vi "std sort simple.vi"(8 "error in":errorcluster, 11 "cycle results cluster IN":T2) -> (0 "error out":errorcluster, 3 "output cluster":T1)   [LabVIEW 2016]
uses:
  controls/cycle results control.ctl
  controls/data control cluster.ctl
panel:
  out "Array 2":dbl[][](array[numeric])
  out "Array":dbl[][][](array[numeric])
  out "element 2":dbl
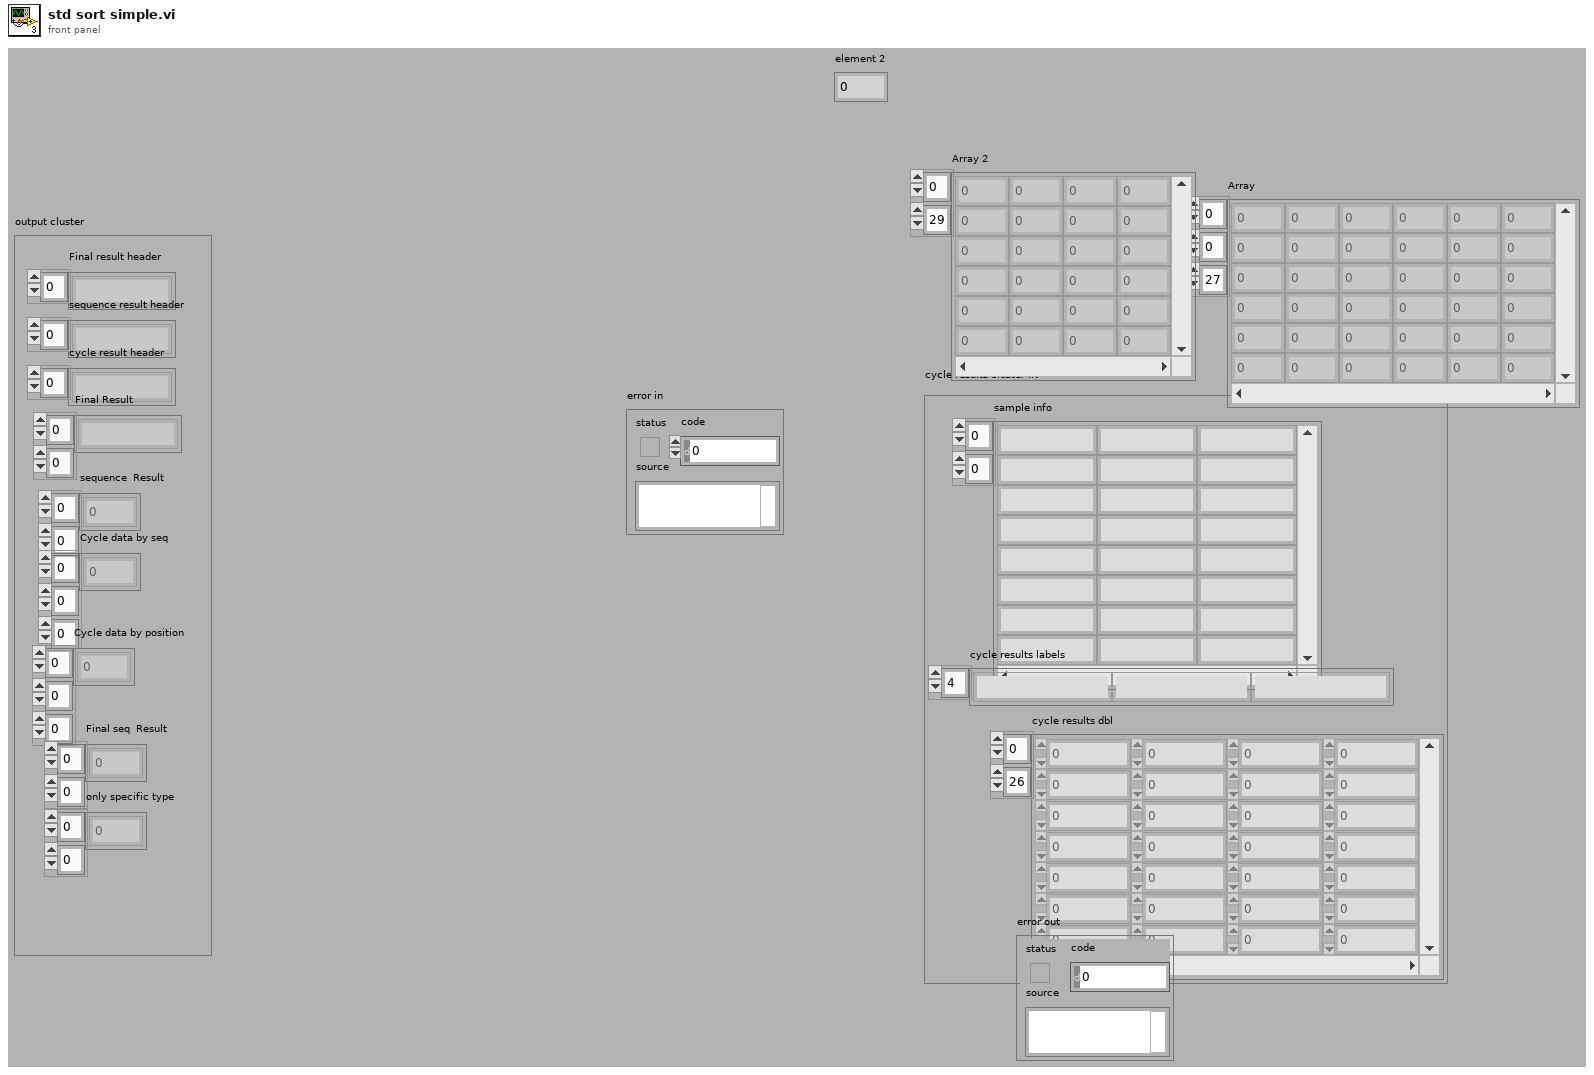
[diagram p1: front panel]
types:
  T1 = typedef "data control cluster.ctl" = cluster{"Final result header":string[], "sequence result header":string[], "cycle result header ":string[], "Final Result":string[][], "sequence  Result":dbl[][], "Cycle data by seq":dbl[][][], "Cycle data by position":dbl[][][], "Final seq  Result":dbl[][], "only specific type":dbl[][]}
  T2 = typedef "cycle results control.ctl" = cluster{"sample info":string[][], "cycle results labels":string[], "cycle results dbl":dbl[][]}
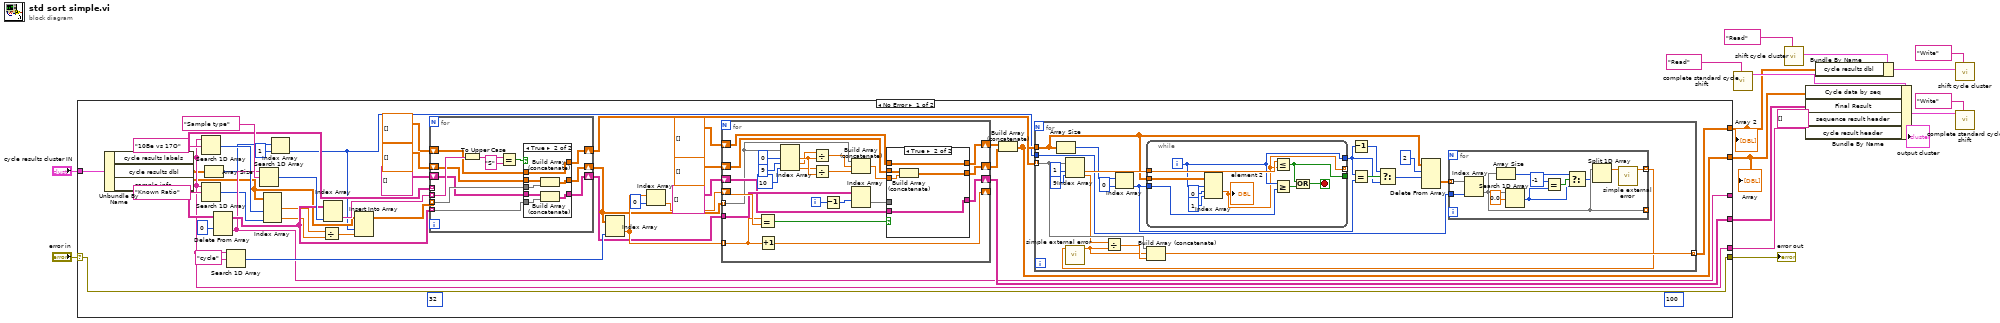
[diagram p0: block diagram]
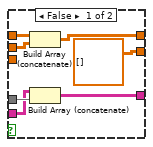
[diagram p2: hidden frame]
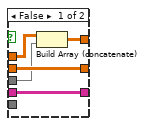
[diagram p3: hidden frame]
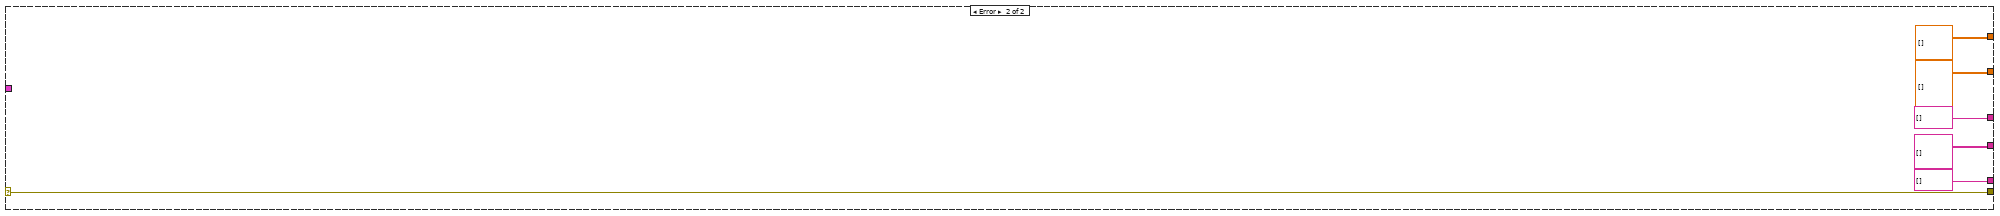
[diagram p4: hidden frame]
diagram:
  n1 = case shown="No Error" "error in" {
    selector: "error in" -> [w57 w164]
    tunnel: "cycle results cluster IN" -> [w35 _]
    tunnel: [w57 w164] -> w14
    tunnel: [w37 string[][] []] -> w7
    tunnel: [w36 string[] [] ("sample info")] -> _
    tunnel: [w19 dbl[][][] []] -> w6
    tunnel: [w32 string[] [] ("cycle results labels")] -> w9
    tunnel: [w17 dbl[][] []] -> w2
    frame No Error {
      (unwired) 32
      (unwired) 100 ("disabled index (col)")
      n2 = Unbundle By Name(w35) -> ("cycle results labels"=w32:string[], "cycle results dbl"=w25:dbl[][], "sample info"=w51:string[][])
      n3 = Search 1D Array(1D array=w32, element="10Be vs 17O") -> (index of element=w31:i32)  [unwired: 1 in]
      n4 = Search 1D Array(1D array=w32, element="Known Ratio") -> (index of element=w30:i32)  [unwired: 1 in]
      n5 = Array Size(array=w25) -> (size(s)=w24:i32[])
      n6 = Delete From Array(array=w51, index (row)=0) -> (deleted portion=w36:string[], array with subset deleted=w50:string[][])  [unwired: 2 in]
      n7 = Search 1D Array(1D array=w32, element="cycle") -> (index of element=w47:i32)  [unwired: 1 in]
      n8 = Search 1D Array(1D array=w36, element="Sample type") -> (index of element=w54:i32)  [unwired: 1 in]
      n9 = Index Array(array=w25, index (col) #1=w31, index (col) #2=w30) -> (element #1=w29:dbl[], element #2=w28:dbl[])  [unwired: 2 in]
      n10 = Index Array(array=w24, index=1) -> (element=w18:i32)
      n11 = Divide(x=w29, y=w28) -> (x/y=w26:dbl[])
      n12 = Index Array(array=w50, index (col)=w54) -> (element=w53:string[])  [unwired: 1 in]
      n13 = Insert Into Array(array=w25, index (col)=w18, new element=w26) -> (w27:dbl[][])  [unwired: 1 in]
      n14 = for {
        tunnel: w51 -> [_] mode=indexing
        tunnel: w27 -> [w142] mode=indexing
        tunnel: w53 -> [w146] mode=indexing
        shift-right: [w141] -> w21
        shift-left: dbl[][] [] -> [w140]
        tunnel: w50 -> [w139] mode=indexing
        shift-right: [w138] -> w39
        shift-left: string[][] [] -> [w137]
        shift-right: [w136] -> w20
        shift-left: dbl[][] [] -> [w135]
        n15 = To Upper Case(1:w146) -> (0:w145:string)
        n16 = Equal?(x=w145, y="S") -> (x = y?=w143:bool)
        n17 = case shown="True" w143 {
          tunnel: w142 -> [w149 w158]
          tunnel: [w151 w157] -> w141
          tunnel: w140 -> [w151 w156]
          tunnel: w139 -> [_ w155]
          tunnel: [w150 w153] -> w138
          tunnel: w137 -> [w150 w154]
          tunnel: [w148 w152] -> w136
          tunnel: w135 -> [w147 w152]
          frame False {
            n18 = Build Array (concatenate)(w147, w149) -> (w148:dbl[][])
          }
          frame True {
            n19 = Build Array (concatenate)(w156, w158) -> (w157:dbl[][])
            n20 = Build Array (concatenate)(w154, w155) -> (w153:string[][])
          }
        }
      }
      n21 = Index Array(array=w21, index (col)=w47) -> (element=w46:dbl[])  [unwired: 1 in]
      n22 = Index Array(array=w46, index=0) -> (element=w40:dbl)
      n23 = for {
        tunnel: w46 -> [w116] mode=indexing
        shift-right: [w115] -> _
        shift-left: w40 -> [w122]
        tunnel: w21 -> [w102] mode=indexing
        shift-right: [w121] -> w43
        shift-left: dbl[][] [] -> [w120]
        shift-right: [w119] -> w42
        shift-left: dbl[][][] [] -> [w118]
        tunnel: w39 -> [w114]
        shift-right: [w112] -> w37
        shift-left: string[][] [] -> [w110]
        i -> [w113]
        n24 = Equal?(x=w116, y=w122) -> (x = y?=w117:bool)
        n25 = Increment(x=w116) -> (x+1=w115:dbl)
        n26 = Index Array(array=w102, index #1=0 ("index"), index #2=9 ("index"), index #3=10 ("index")) -> (element #1=w105:dbl, element #2=w103:dbl, element #3=w104:dbl)
        n27 = Divide(x=w103, y=w105) -> (x/y=w101:dbl)
        n28 = Divide(x=w104, y=w105) -> (x/y=w100:dbl)
        n29 = Decrement(x=w113) -> (x-1=w109:i32)
        n30 = Build Array (concatenate)(w102, w101, w100) -> (w99:dbl[])
        n31 = Index Array(array=w114, index (row)=w109) -> (element=w111:string[])  [unwired: 1 in]
        n32 = case shown="True" w117 {
          tunnel: w99 -> [_ w134]
          tunnel: [dbl[][] [] w133] -> w121
          tunnel: w120 -> [w129 w132]
          tunnel: [w128 w131] -> w119
          tunnel: w118 -> [w127 w131]
          tunnel: [w123 w130] -> w112
          tunnel: w111 -> [w125 _]
          tunnel: w110 -> [w124 w130]
          frame False {
            n33 = Build Array (concatenate)(w127, w129) -> (w128:dbl[][][])
            n34 = Build Array (concatenate)(w124, w125) -> (w123:string[][])
          }
          frame True {
            n35 = Build Array (concatenate)(w132, w134) -> (w133:dbl[][])
          }
        }
      }
      n36 = Build Array (concatenate)(w42, w43) -> (w19:dbl[][][])
      n37 = for {
        tunnel: w20 -> [w68] mode=indexing
        tunnel: w19 -> [w72]
        tunnel: w18 -> [w69]
        tunnel: [w67] -> w17 mode=indexing
        n38 = Array Size(array=w72) -> (size(s)=w74:i32[])
        n39 = Index Array(array=w68, index #1=1 ("index"), index #2=9 ("index")) -> (element #1=w75:dbl, element #2=w64:dbl)
        n40 = Index Array(array=w74, index=0) -> (element=w63:i32)
        n41 = while {
          tunnel: w72 -> [w98]
          tunnel: w75 -> [w95]
          tunnel: w63 -> [w94]
          tunnel: [w91] -> w60
          tunnel: [w90] -> _
          tunnel: [w89] -> _ mode=indexing
          i -> [w91]
          stop <- w92 stop-if-true
          n42 = Index Array(array=w98, index (dim 0)=w91, index (dim 1)=0 ("disabled index (row)"), index (dim 2)=1 ("disabled index (col)")) -> (element=w89:dbl)
          "element 2" <- w89
          n43 = Less Or Equal?(x=w95, y=w89) -> (x <= y?=w90:bool)
          n44 = Greater Or Equal?(x=w91, y=w94) -> (x >= y?=w93:bool)
          n45 = Or(x=w90, y=w93) -> (x .or. y?=w92:bool)
        }
        n46 = Decrement(x=w60) -> (x-1=w61:i32)
        n47 = Equal?(x=w60, y=w63) -> (x = y?=w62:bool)
        n48 = Select(t=w61, s=w62, f=w60) -> (s? t:f=w59:i32)
        n49 = Delete From Array(array=w72, length=2, index (dim 0)=w59) -> (deleted portion=w70:dbl[][][])  [unwired: 2 in, 1 out]
        n50 = for {
          tunnel: w70 -> [w88] mode=indexing
          tunnel: w69 -> [w87]
          tunnel: [w81] -> _ mode=indexing
          tunnel: [w86] -> w58 mode=indexing
          n51 = Index Array(array=w88, index (col)=w87) -> (element=w81:dbl[])  [unwired: 1 in]
          n52 = Array Size(array=w81) -> (size(s)=w80:i32)
          n53 = Search 1D Array(1D array=w81, element=0.0) -> (index of element=w79:i32)  [unwired: 1 in]
          n54 = Equal?(x=-1, y=w79) -> (x = y?=w82:bool)
          n55 = Select(t=w80, s=w82, f=w79) -> (s? t:f=w78:i32)
          n56 = Split 1D Array(array=w81, index=w78) -> (first subarray=w84:dbl[])  [unwired: 1 out]
          n57 = call "simple external error.vi"("cycle results"=w84) -> ("Sequence result"=w86:dbl)  [unwired: 7 in, 3 out]
        }
        n58 = call "simple external error.vi"("cycle results"=w58) -> ("Sequence result"=w65:dbl)  [unwired: 7 in, 3 out]
        n59 = Divide(x=w64, y=w65) -> (x/y=w66:dbl)
        n60 = Build Array (concatenate)(w68, w65, w66) -> (w67:dbl[])
      }
    }
    frame Error {
    }
  }
  "error out" <- w14
  "Array" <- w6
  "Array 2" <- w2
  n61 = call "complete standard cycle shift.vi"("read write shift"="Read") -> ("DATA CLUSTER out"=w12:T1)  [unwired: 9 in, 1 out]
  n62 = call "shift cycle cluster.vi"("read write shift"="Read") -> ("cycle results cluster out"=w3:T2)  [unwired: 9 in, 1 out]
  n63 = Bundle By Name(cluster=w12, "Cycle data by seq"=w6, "Final Result"=w7, "sequence result header"=string[] [], "cycle result header"=w9) -> (w13:T1)
  "output cluster" <- w13
  n64 = Bundle By Name(cluster=w3, "cycle results dbl"=w2) -> (w1:T2)
  n65 = call "shift cycle cluster.vi"("read write shift"="Write", "cycle results cluster In"=w1) -> ()  [unwired: 8 in, 2 out]
  n66 = call "complete standard cycle shift.vi"("read write shift"="Write", "DATA CLUSTER in"=w13) -> ()  [unwired: 8 in, 2 out]
